vi "microFPGA_version_read_addr_200_ctrl.vi"(0 "VISA resource name":refnum<visa-resource-name>="COM118", 11 "error in (no error)":errorcluster) -> (4 "VISA resource name 2":refnum<visa-resource-name>="COM118", 6 "Version":u16=3, 15 "error out":errorcluster={"status"=FALSE, "code"=1073676294, "source"="VISA Read in read_string.vi->microFPGA_version_read_addr_100_ctrl.vi->test microFPGA VIs.vi"})   [LabVIEW 2018]
panel:
  out "mode read string answer":string
  out "mode read string":string
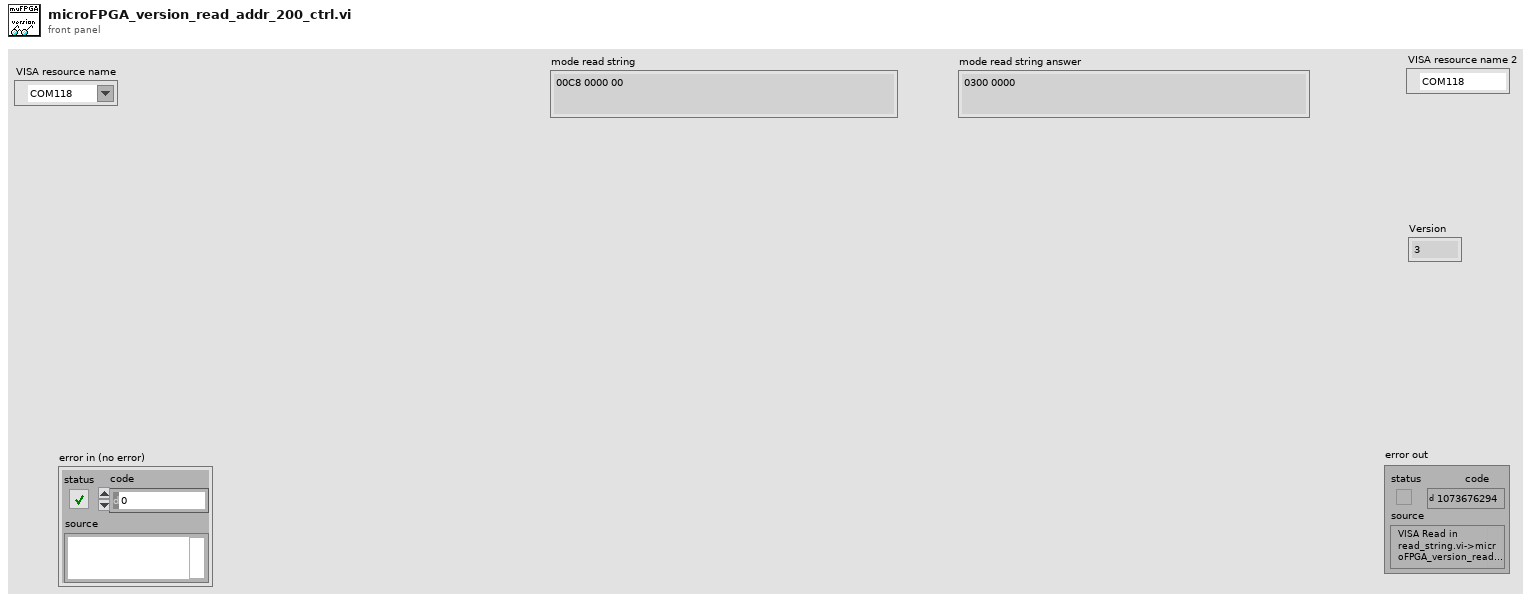
[diagram p1: front panel]
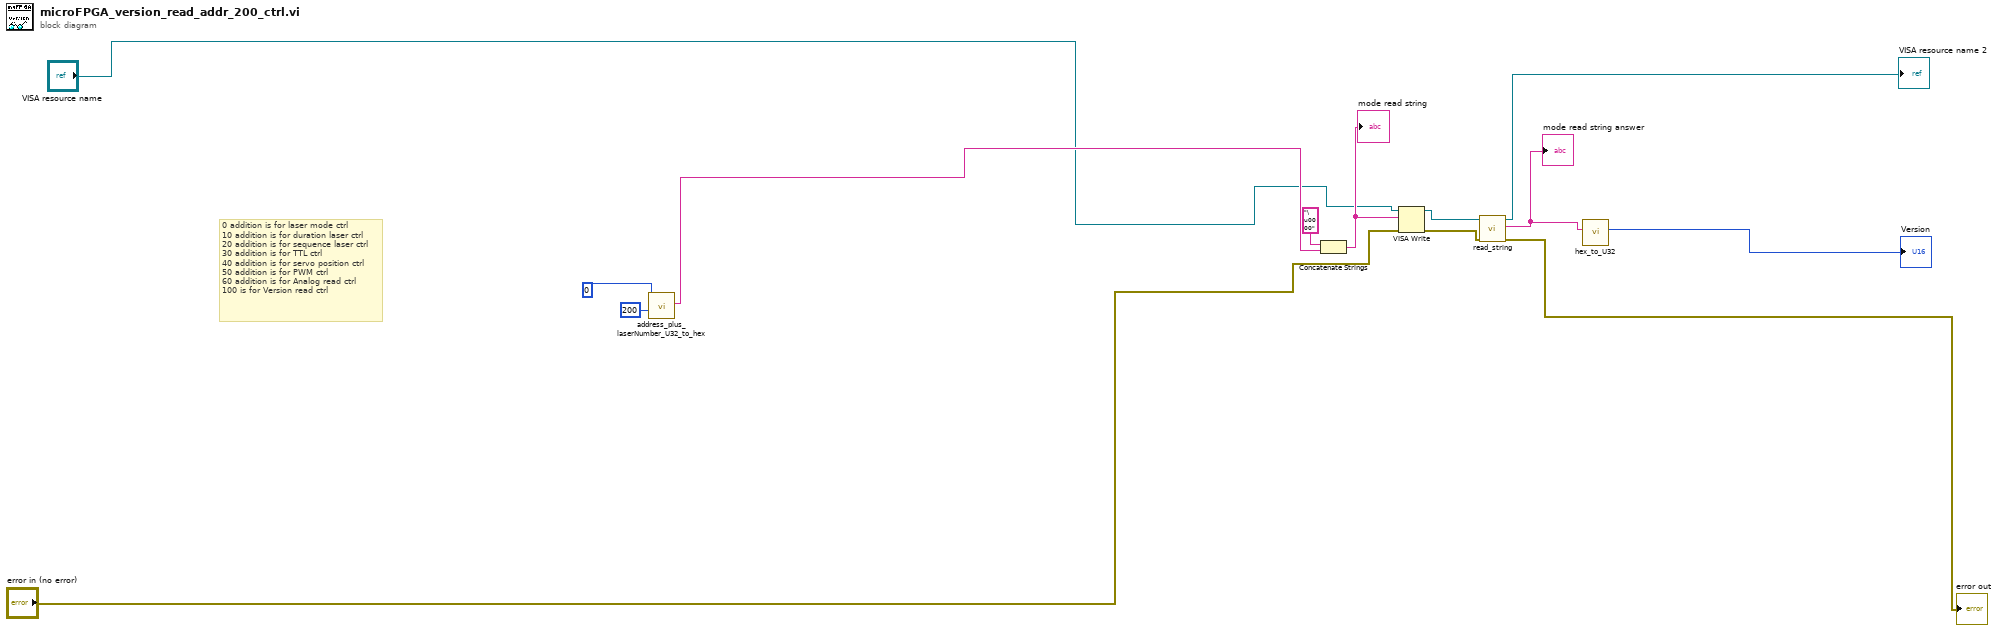
[diagram p0: block diagram]
diagram:
  # "0 addition is for laser mode ctrl\n10 addition is for duration laser ctrl\n20 addition is for sequence laser ctrl\n30 addition is for TTL ctrl\n40 addition is for servo position ctrl\n50 addition is for PWM ctrl\n60 addition is for Analog read ctrl\n100 is for Version read ctrl"
  n1 = call "address_plus_laserNumber_U32_to_hex.vi"("adress offset"=u32 200, "y 3"=u32 0) -> ("string 5"=w8:string)  [unwired: 8 in]
  n2 = Concatenate Strings("\u0000" ("string"), w8) -> (w7:string)
  "mode read string" <- w7
  n3 = VISA Write(VISA resource name="VISA resource name", write buffer=w7, error in (no error)="error in (no error)") -> (VISA resource name out=w6:refnum<visa-resource-name>, error out=w5:errorcluster)  [unwired: 1 out]
  n4 = call "read_string.vi"("error in (no error)"=w5, "VISA resource name 2"=w6) -> ("error out"=→"error out":errorcluster, "read buffer"=w3:string, "VISA resource name"=→"VISA resource name 2":refnum<visa-resource-name>)  [unwired: 7 in]
  "mode read string answer" <- w3
  n5 = call "hex_to_U32.vi"("hex"=w3) -> ("U32"=→"Version":u32)  [unwired: 9 in]
